vi "Set_Data.vi"(8 "error in (no error)":errorcluster caption="entrée d'erreur (pas d'erreur)", 11 "Firebase Benches en entrée":refnum<class "Firebase Scan.lvclass">) -> (0 "error out":errorcluster caption="sortie d'erreur", 3 "Firebase Benches en sortie":refnum<class "Firebase Scan.lvclass">)   [LabVIEW 2020, in "Library Instrument & Equipement.lvlib" / "Library FireBase.lvlib" / "Firebase Scan.lvclass"]
doc: "Create New document\nPlease initialise the following values\n - Name BDD\n - Document\n - API Key"
uses:
  Firebase Scan.lvclass
  C:/Users/ngarcin/OneDrive - Altyor/Standard TB/Class/Firebase/Source/Firebase Altyor/Firebase Altyor.lvclass
  C:/Users/ngarcin/OneDrive - Altyor/Standard TB/Class/Firebase/Source/Firebase Driver/Firebase Driver.lvclass
  Firebase Scan.lvclass/Firebase Scan.ctl
  Firebase Altyor/Firebase Altyor.lvclass
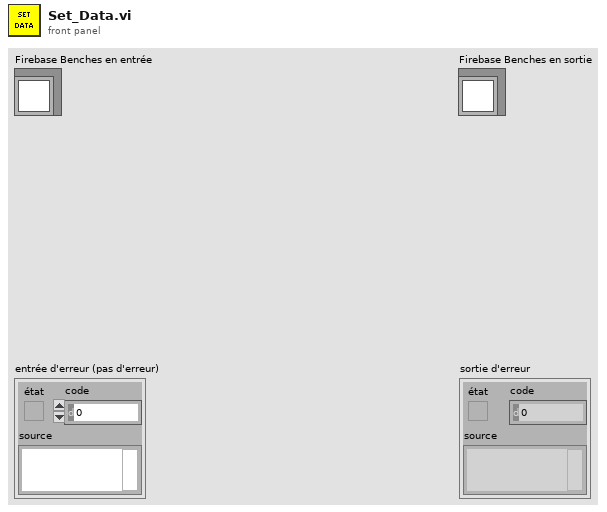
[diagram p1: front panel]
types:
  T1 = cluster{"fields":cluster{"Result":cluster{"booleanValue":bool}, "CreationDate":cluster{"timestampValue":string}, "Batch":cluster{"stringValue":string}, "SerialNumber":cluster{"stringValue":string}, "EndOfProduction":cluster{"timestampValue":string}, "FW_Version":cluster{"mapValue":cluster{"fields":cluster{"Bootloader":cluster{"mapValue":cluster{"fields":cluster{"File_Name":cluster{"stringValue":string}, "Version":cluster{"mapValue":cluster{"fields":cluster{"Major":cluster{"stringValue":string}, "Minor":cluster{"stringValue":string}}}}, "Checksum":cluster{"stringValue":string}}}}, "SoftDevice":cluster{"mapValue":cluster{"fields":cluster{"File_Name":cluster{"stringValue":string}, "Version":cluster{"mapValue":cluster{"fields":cluster{"Major":cluster{"stringValue":string}, "Minor":cluster{"stringValue":string}}}}, "Checksum":cluster{"stringValue":string}}}}, "DFU":cluster{"mapValue":cluster{"fields":cluster{"File_Name":cluster{"stringValue":string}, "Version":cluster{"mapValue":cluster{"fields":cluster{"Major":cluster{"stringValue":string}, "Minor":cluster{"stringValue":string}}}}, "Checksum":cluster{"stringValue":string}}}}}}}, "PartNumber":cluster{"stringValue":string}, "OrderNumber":cluster{"stringValue":string}, "Operator":cluster{"stringValue":string}, "Deleted":cluster{"booleanValue":bool}}}
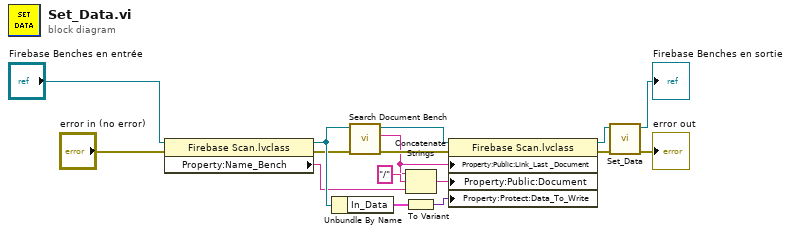
[diagram p0: block diagram]
diagram:
  n1 = property class="Firebase Scan.lvclass"(reference="Firebase Benches en entrée", error in="error in (no error)") -> (reference out=w4:refnum<class "Firebase Scan.lvclass">, error out=w1:errorcluster, "Property:Name_Bench"=w3:string)
  n2 = Unbundle By Name(w4) -> ("In_Data"=w12:T1)
  n3 = call "Search Document Bench.vi"("entrée d'erreur (pas d'erreur)"=w1, "Firebase Altyor en entrée"=w4) -> ("sortie d'erreur"=w9:errorcluster, "Source"=w6:string, "Firebase Altyor en sortie"=w10:refnum<class "Firebase Scan.lvclass">)  [unwired: 7 in]
  n4 = Concatenate Strings(w6, "/" ("chaîne"), w3) -> (w7:string)
  n5 = To Variant(anything=w12) -> (Variant=w8:variant)
  n6 = property class="Firebase Scan.lvclass"(reference=w10, error in=w9, "Property:Public:Link_Last _Document"=w6, "Property:Public:Document"=w7, "Property:Protect:Data_To_Write"=w8) -> (reference out=w14:refnum<class "Firebase Scan.lvclass">, error out=w13:errorcluster)
  n7 = call-parent "Set_Data.vi"("error in (no error)"=w13, "Firebase Altyor en entrée"=w14) -> ("error out"=→"error out":errorcluster, "Firebase Altyor en sortie"=→"Firebase Benches en sortie":refnum<class "Firebase Scan.lvclass">)  [unwired: 8 in]
